vi "About.vi"(0 "Revision Number":string) -> ()   [LabVIEW 2010]
doc: "Use this template to create a dialog box. This template polls the state of the buttons on the front panel and does not use events. Use the Dialog Using Events template (not available in Base package) to create a dialog box with event handling."
panel:
  in  "OK":bool
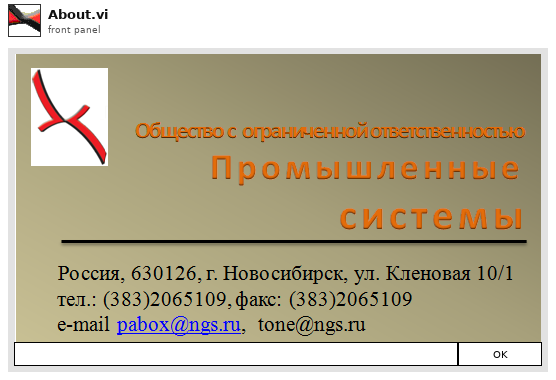
[diagram p1: front panel]
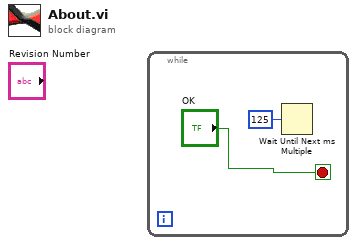
[diagram p0: block diagram]
diagram:
  n1 = while {
    stop <- "OK" stop-if-true
    n2 = Wait Until Next ms Multiple(millisecond multiple=u32 125) -> ()  [unwired: 1 out]
  }
